vi "Intake Controller.vi"(8 "error in":errorcluster) -> ()   [LabVIEW 2020]
doc: "This VI executes continuously carrying out the current operation and responding to updates or new operations. It will often contain the timing or control code that is difficult to place directly in TeleOp. This VI generally opens all sensors and motors and isolates the rest of the robot code from knowing how the operations are carried out."
uses:
  <vilib>/Rock Robotics/WPI/Framework/Completion Status.ctl
  Intake Setpoints.ctl
  Intake Operations.ctl
  <vilib>/Rock Robotics/WPI/Solenoid/WPI_SolenoidValue.ctl
  <vilib>/Rock Robotics/WPI/Solenoid/WPI_SolenoidSetEnum.vi
  <vilib>/Rock Robotics/WPI/Solenoid/WPI_SolenoidGetEnum.vi
  <vilib>/Rock Robotics/Network Tables/NT Write Boolean.vi
panel:
  in  "Interactive Values":T1
  out "Current\nCmd":string
  in  "Buttons":cluster{"Execute Cmd":bool, "Abort Cmd":bool}
  out "Command Timing":cluster{"Start Time (ms)":u32, "Iterations":i32}
  out "Status":T3
  # "Tip: It may be helpful to observe inputs and sensor values.\nYou may also want to display tuning or debugging controls."
  # "Interactive Command: You may fill in the settings for a command\nand schedule it with the Execute button. You can observe and abort\nany command while fine tuning the code for the controller."
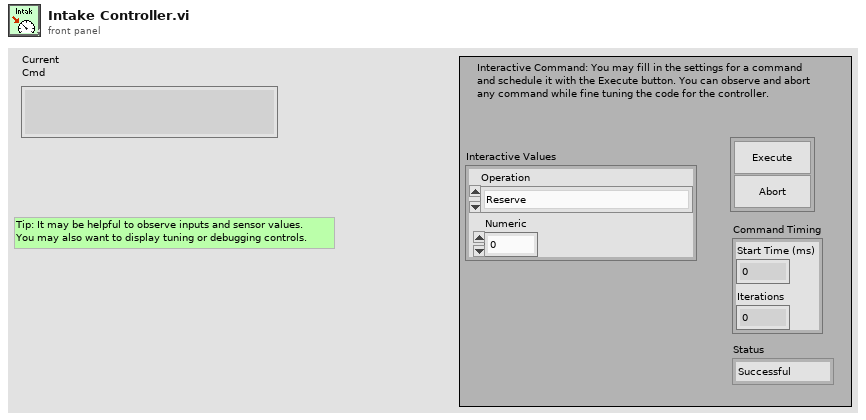
[diagram p1: front panel]
types:
  T1 = typedef "Intake Setpoints.ctl" = cluster{"Operation":T2, "Numeric":dbl}
  T2 = typedef "Intake Operations.ctl" = enum16{"Reserve", "Read Current", "Immediate", "Retract", "Extend", "Feed"}
  T3 = typedef "Completion Status.ctl" = enum16{"Successful", "Aborted", "Incomplete"}
  T4 = typedef "Command Status Info.ctl" = cluster{"Name":string, "Status":T3, "notifier out":T5}
  T5 = typedef "Completion Notifier.ctl" = refnum<notifier>
  T6 = cluster{"Current Command":T1, "Command Timing":cluster{"Start Time (ms)":u32, "Iterations":i32}, "Command Arguments":cluster{"Command Info":T4, "Description":string, "Default Command":T1, "queue out":refnum<queue>, "Subsystem Name":string}}
  T7 = typedef "WPI_SolenoidValue.ctl" = enum16{"Off", "On", "Forward", "Reverse"}
  T8 = typedef "WPI_SolenoidDevRef.ctl" = cluster{"DevStatus":errorcluster, "Pneumatics Control Module":u8, "Forward Solenoid Channel":T9, "Reverse Solenoid Channel":T9}
  T9 = typedef "WPI_SolenoidChannel.ctl" = enum8{"Solenoid 0", "Solenoid 1", "Solenoid 2", "Solenoid 3", "Solenoid 4", "Solenoid 5", "Solenoid 6", "Solenoid 7", "Solenoid 8", "Solenoid 9", "Solenoid 10", "Solenoid 11", "Solenoid 12", "Solenoid 13", "Solenoid 14", "Solenoid 15", "Invalid"}
  T10 = typedef "WPI_MotorControlDeviceRef.ctl" = cluster{"DeviceStatus":errorcluster, "Type":T11, "PWM":cluster{"PWM Channel":T12, "DeadBand":T13}, "CAN":cluster{"Device Number":u8, "SetOutput VI Ref":variant, "GetOutput VI Ref":variant, "Enable VI Ref":variant, "Disable VI Ref":variant, "Data":variant}, "Invert":bool, "DIO PWM":cluster{"PWM \"Enable\" Channel":T12, "DIOChannel":T14, "PWM Rate":dbl}}
  T11 = typedef "WPI_MotorControlType.ctl" = enum16{"PWM", "CAN", "DIO PWM"}
  T12 = typedef "FPGA_DIOPWMChannel.ctl" = enum8{"PWM 0", "PWM 1", "PWM 2", "PWM 3", "PWM 4", "PWM 5", "PWM 6", "PWM 7", "PWM 8", "PWM 9", "PWM MXP 0", "PWM MXP 1", "PWM MXP 2", "PWM MXP 3", "PWM MXP 4", "PWM MXP 5", "PWM MXP 6", "PWM MXP 7", "PWM MXP 8", "PWM MXP 9", "Invalid"}
  T13 = typedef "WPI_PWMDeadband.ctl" = cluster{"Name":string, "maxPositivePwm":i32, "minPositivePwm":i32, "centerPwm":i32, "maxNegativePwm":i32, "minNegativePwm":i32, "angularRange":u16}
  T14 = typedef "FPGA_DIOChannel.ctl" = enum8{"DIO 0", "DIO 1", "DIO 2", "DIO 3", "DIO 4", "DIO 5", "DIO 6", "DIO 7", "DIO 8", "DIO 9", "DIO MXP 0", "DIO MXP 1", "DIO MXP 2", "DIO MXP 3", "DIO MXP 4", "DIO MXP 5", "DIO MXP 6", "DIO MXP 7", "DIO MXP 8", "DIO MXP 9", "DIO MXP 10", "DIO MXP 11", "DIO MXP 12", "DIO MXP 13", "DIO MXP 14", "DIO MXP 15", "SPI Port CS1", "SPI Port CS2", "SPI Port CS3", "SPI Port MISO", "SPI Port MOSI", "Invalid"}
  T15 = typedef "WPI_DigitalInputDevRef.ctl" = cluster{"DevStatus":errorcluster, "DIO Channel":T14}
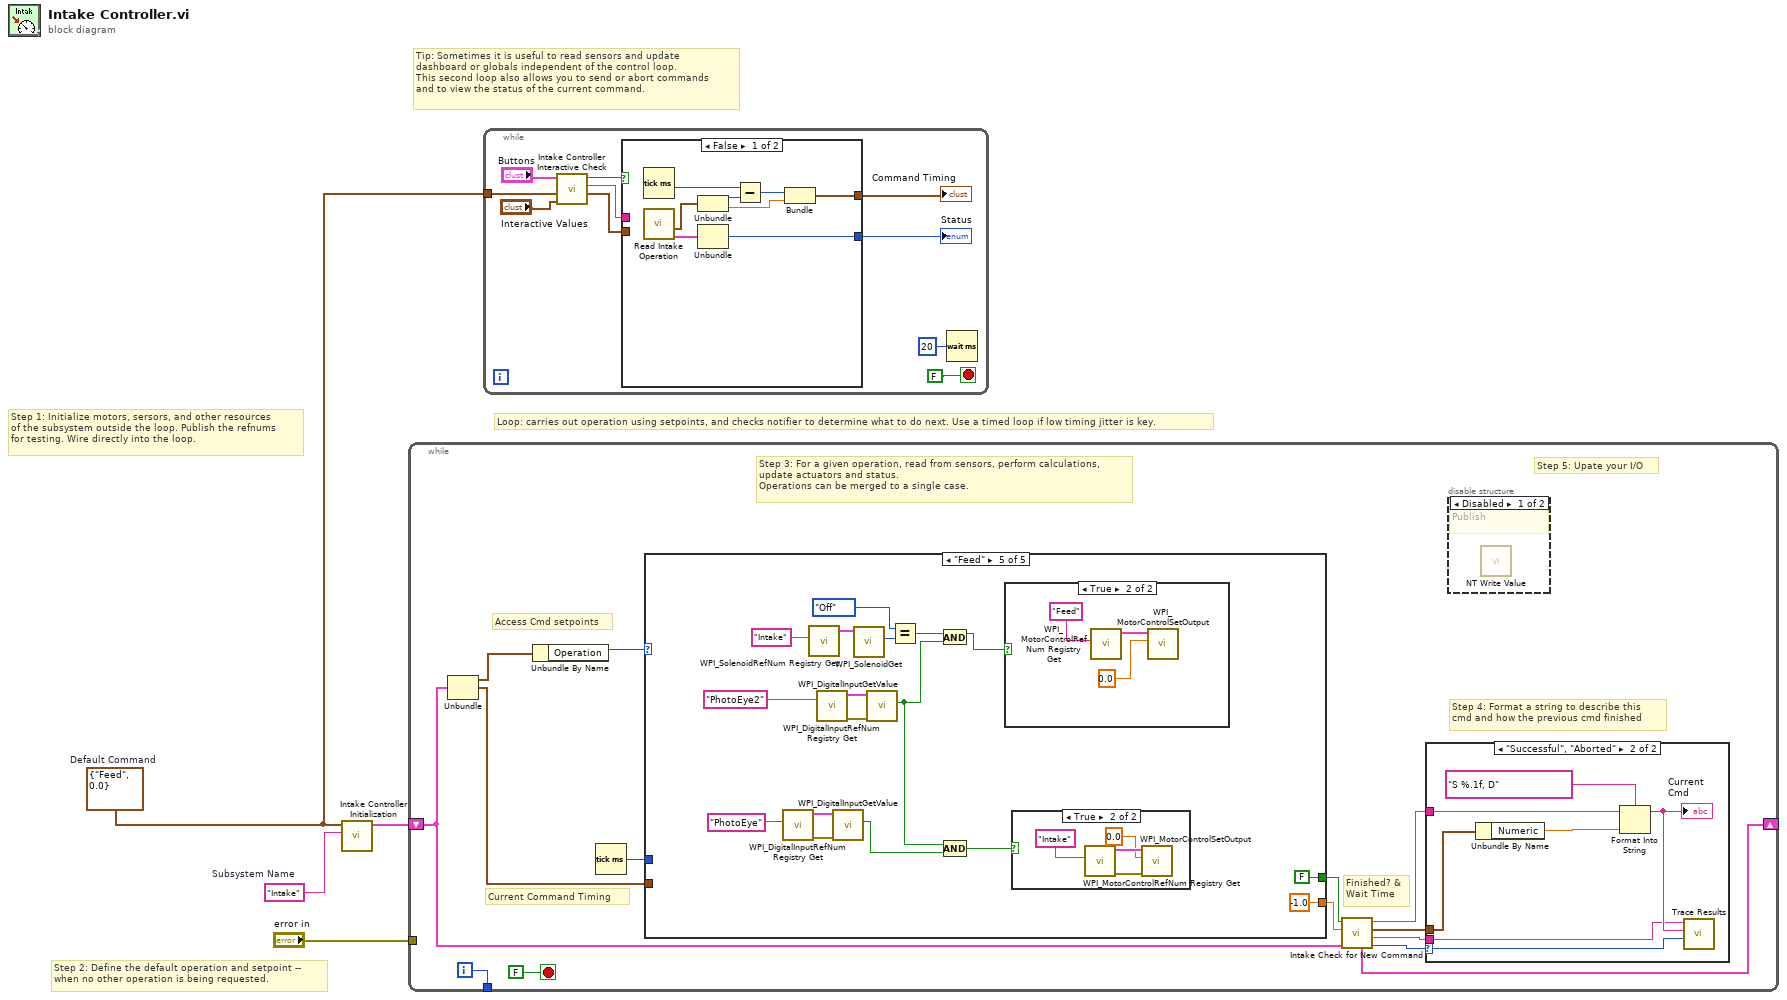
[diagram p0: block diagram]
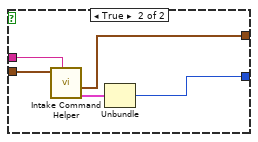
[diagram p2: hidden frame]
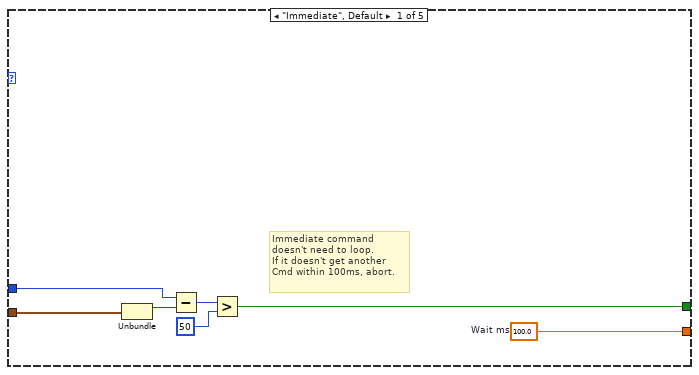
[diagram p5: hidden frame]
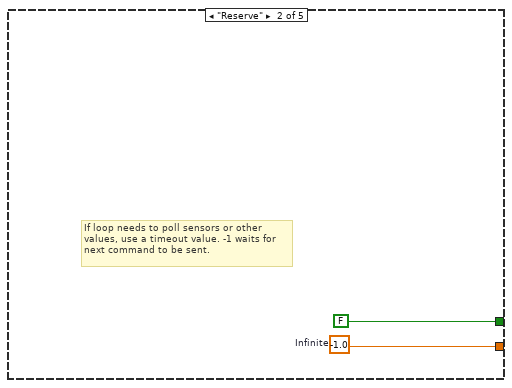
[diagram p6: hidden frame]
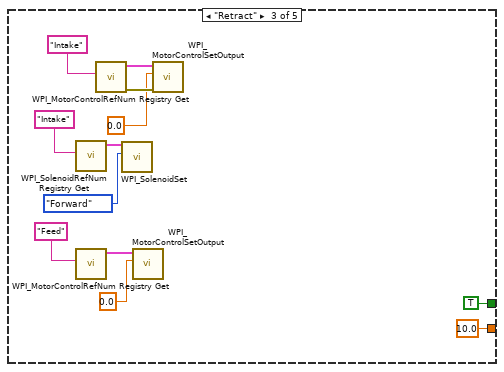
[diagram p7: hidden frame]
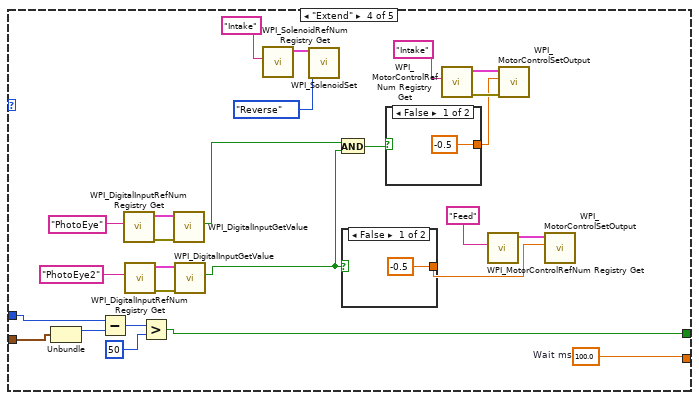
[diagram p8: hidden frame]
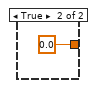
[diagram p9: hidden frame]
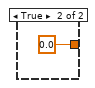
[diagram p10: hidden frame]
diagram:
  w1 = T1 {"Operation"=enum."Feed", "Numeric"=0.0}  # Default Command
  w2 = "Intake"  # Subsystem Name
  # "Tip: Sometimes it is useful to read sensors and update\ndashboard or globals independent of the control loop.\nThis second loop also allows you to send or abort commands\nand to view the status of the current command."
  # "Step 2: Define the default operation and setpoint --\nwhen no other operation is being requested."
  # "Step 1: Initialize motors, sersors, and other resources\nof the subsystem outside the loop. Publish the refnums\nfor testing. Wire directly into the loop."
  # "Loop: carries out operation using setpoints, and checks notifier to determine what to do next. Use a timed loop if low timing jitter is key."
  n1 = call "Intake Controller Initialization.vi"("Subsystem Name"=w2, "Default Command"=w1) -> ("Current Command"=w3:T6)  [unwired: 9 in]
  n2 = while {
    shift-right: [w12] -> _
    shift-left: w3 -> [w5]
    tunnel: [w17] -> _
    tunnel: "error in" -> [_]
    i -> [w17]
    stop <- FALSE stop-if-true
    # "Step 5: Upate your I/O"
    # "Step 4: Format a string to describe this\ncmd and how the previous cmd finished"
    # "Current Command Timing"
    # "Access Cmd setpoints"
    # "Finished? &\nWait Time"
    # "Step 3: For a given operation, read from sensors, perform calculations,\nupdate actuators and status.\nOperations can be merged to a single case."
    n3 = Unbundle(w5) -> ("Current Command"=w16:T1, "Command Timing"=w13:cluster{"Start Time (ms)":u32, "Iterations":i32})  [unwired: 1 out]
    n4 = Unbundle By Name(w16) -> ("Operation"=w15:T2)
    n5 = Tick Count (ms)() -> (millisecond timer value=w14:u32)
    n6 = case shown="\"Feed\"" w15 {
      tunnel: [w32 w34 10.0 ("Wait ms") w47 -1.0 ("Wait ms")] -> w10
      tunnel: [w26 FALSE ("ignore previous (F)") TRUE ("ignore previous (F)") w48 FALSE ("ignore previous (F)")] -> w11
      tunnel: w13 -> [w28 _ _ w49 _]
      tunnel: w14 -> [w27 _ _ w50 _]
      frame "Immediate", Default {
        w32 = 100.0  # Wait ms
        # "Immediate command\ndoesn't need to loop.\nIf it doesn't get another\nCmd within 100ms, abort."
        n7 = Unbundle(w28) -> ("Start Time (ms)"=w31:u32)  [unwired: 1 out]
        n8 = Subtract(x=w27, y=w31) -> (x-y=w30:u32)
        n9 = Greater?(x=w30, y=u8 50 ("Left Motor")) -> (0:w26:bool)
      }
      frame "Reserve" {
        w34 = -1.0  # Infinite
        # "If loop needs to poll sensors or other\nvalues, use a timeout value. -1 waits for\nnext command to be sent."
      }
      frame "Retract" {
        n10 = call <vilib>:"WPI_SolenoidRefNum Registry Get.vi"("refnum name"="Intake") -> ("SolenoidDevRef"=w45:T8)  [unwired: 9 in, 1 out]
        n11 = call <vilib>:"WPI_MotorControlRefNum Registry Get.vi"("refnum name"="Feed") -> ("MotorControlDevRef"=w46:T10)  [unwired: 9 in, 1 out]
        n12 = call <vilib>:"WPI_MotorControlRefNum Registry Get.vi"("refnum name"="Intake") -> ("error out"=w44:errorcluster, "MotorControlDevRef"=w43:T10)  [unwired: 9 in]
        n13 = call-poly <vilib>:"WPI_SolenoidSet.vi"("Value"=WPI_SolenoidValue."Forward", "SolenoidDevRef"=w45) -> ()  [unwired: 8 in, 2 out]
        n14 = call <vilib>:"WPI_MotorControlSetOutput.vi"("Output"=0.0, "MotorControlDevRef"=w46) -> ()  [unwired: 7 in, 3 out]
        n15 = call <vilib>:"WPI_MotorControlSetOutput.vi"("error in (no error)"=w44, "Output"=0.0, "MotorControlDevRef"=w43) -> ()  [unwired: 6 in, 3 out]
      }
      frame "Extend" {
        w47 = 100.0  # Wait ms
        n16 = Unbundle(w49) -> ("Start Time (ms)"=w53:u32)  [unwired: 1 out]
        n17 = Subtract(x=w50, y=w53) -> (x-y=w52:u32)
        n18 = call <vilib>:"WPI_DigitalInputRefNum Registry Get.vi"("refnum name"="PhotoEye") -> ("error out"=w63:errorcluster, "DigitalInputDevRef"=w62:T15)  [unwired: 9 in]
        n19 = call <vilib>:"WPI_DigitalInputRefNum Registry Get.vi"("refnum name"="PhotoEye2") -> ("error out"=w61:errorcluster, "DigitalInputDevRef"=w60:T15)  [unwired: 9 in]
        n20 = Greater?(x=w52, y=u8 50 ("Left Motor")) -> (0:w48:bool)
        n21 = call <vilib>:"WPI_DigitalInputGetValue.vi"("error in (no error)"=w63, "DigitalInputDevRef"=w62) -> ("Value"=w57:bool)  [unwired: 7 in, 2 out]
        n22 = call <vilib>:"WPI_DigitalInputGetValue.vi"("error in (no error)"=w61, "DigitalInputDevRef"=w60) -> ("Value"=w56:bool)  [unwired: 7 in, 2 out]
        n23 = call <vilib>:"WPI_SolenoidRefNum Registry Get.vi"("refnum name"="Intake") -> ("SolenoidDevRef"=w72:T8)  [unwired: 9 in, 1 out]
        n24 = call-poly <vilib>:"WPI_SolenoidSet.vi"("Value"=WPI_SolenoidValue."Reverse", "SolenoidDevRef"=w72) -> ()  [unwired: 8 in, 2 out]
        n25 = And(x=w57, y=w56) -> (x .and. y?=w66:bool)
        n26 = case shown="False" w56 {
          tunnel: [-0.5 ("Output") 0.0 ("Output")] -> w55
          frame False {
          }
          frame True {
          }
        }
        n27 = case shown="False" w66 {
          tunnel: [-0.5 ("Output") 0.0 ("Output")] -> w54
          frame False {
          }
          frame True {
          }
        }
        n28 = call <vilib>:"WPI_MotorControlRefNum Registry Get.vi"("refnum name"="Intake") -> ("error out"=w68:errorcluster, "MotorControlDevRef"=w67:T10)  [unwired: 9 in]
        n29 = call <vilib>:"WPI_MotorControlRefNum Registry Get.vi"("refnum name"="Feed") -> ("MotorControlDevRef"=w65:T10)  [unwired: 9 in, 1 out]
        n30 = call <vilib>:"WPI_MotorControlSetOutput.vi"("error in (no error)"=w68, "Output"=w54, "MotorControlDevRef"=w67) -> ()  [unwired: 6 in, 3 out]
        n31 = call <vilib>:"WPI_MotorControlSetOutput.vi"("Output"=w55, "MotorControlDevRef"=w65) -> ()  [unwired: 7 in, 3 out]
      }
      frame "Feed" {
        n32 = call <vilib>:"WPI_DigitalInputRefNum Registry Get.vi"("refnum name"="PhotoEye") -> ("error out"=w83:errorcluster, "DigitalInputDevRef"=w82:T15)  [unwired: 9 in]
        n33 = call <vilib>:"WPI_SolenoidRefNum Registry Get.vi"("refnum name"="Intake") -> ("SolenoidDevRef"=w92:T8)  [unwired: 9 in, 1 out]
        n34 = call <vilib>:"WPI_DigitalInputRefNum Registry Get.vi"("refnum name"="PhotoEye2") -> ("error out"=w88:errorcluster, "DigitalInputDevRef"=w87:T15)  [unwired: 9 in]
        n35 = call <vilib>:"WPI_DigitalInputGetValue.vi"("error in (no error)"=w83, "DigitalInputDevRef"=w82) -> ("Value"=w80:bool)  [unwired: 7 in, 2 out]
        n36 = call-poly <vilib>:"WPI_SolenoidGet.vi"("SolenoidDevRef"=w92) -> ("Value"=w93:T7)  [unwired: 8 in, 2 out]
        n37 = call <vilib>:"WPI_DigitalInputGetValue.vi"("error in (no error)"=w88, "DigitalInputDevRef"=w87) -> ("Value"=w79:bool)  [unwired: 7 in, 2 out]
        n38 = Equal?(x=WPI_SolenoidValue."Off", y=w93) -> (x = y?=w78:bool)
        n39 = And(x=w78, y=w79) -> (x .and. y?=w89:bool)
        n40 = Compound Arithmetic op=AND(w79, w80) -> (w77:bool)
        n41 = case shown="True" w89 {
          frame False {
          }
          frame True {
            n42 = call <vilib>:"WPI_MotorControlRefNum Registry Get.vi"("refnum name"="Feed") -> ("MotorControlDevRef"=w100:T10)  [unwired: 9 in, 1 out]
            n43 = call <vilib>:"WPI_MotorControlSetOutput.vi"("Output"=0.0, "MotorControlDevRef"=w100) -> ()  [unwired: 7 in, 3 out]
          }
        }
        n44 = case shown="True" w77 {
          frame False {
          }
          frame True {
            n45 = call <vilib>:"WPI_MotorControlRefNum Registry Get.vi"("refnum name"="Intake") -> ("error out"=w96:errorcluster, "MotorControlDevRef"=w97:T10)  [unwired: 9 in]
            n46 = call <vilib>:"WPI_MotorControlSetOutput.vi"("error in (no error)"=w96, "Output"=0.0, "MotorControlDevRef"=w97) -> ()  [unwired: 6 in, 3 out]
          }
        }
      }
    }
    n47 = call "Intake Check for New Command.vi"("Current Command"=w5, "Wait time (ms)"=w10, "Finished?"=w11) -> ("Completion"=w6:T3, "Subsystem Name"=w7:string, "Current Command"=w8:T1, "Initial Trace String"=w9:string, "NextCommand"=w12:T6)  [unwired: 4 in]
    n48 = case shown="\"Successful\", \"Aborted\"" w6 {
      selector: w6 -> [_ w25]
      tunnel: w9 -> [_ w21]
      tunnel: w8 -> [_ w22]
      tunnel: w7 -> [_ w19]
      frame "Incomplete", Default {
        # "Continuing current command"
      }
      frame "Successful", "Aborted" {
        # "Report and setup for next command"
        n49 = Unbundle By Name(w22) -> ("Numeric"=w24:dbl)
        n50 = Format Into String(format string="S %.1f, D", initial string=w21, w24) -> (resulting string=w20:string)  [unwired: 1 in, 1 out]
        "Current\nCmd" <- w20
        n51 = call <vilib>:"Trace Results.vi"("Status of previous command"=w25, "Description"=w20, "Subsystem"=w19) -> ()  [unwired: 9 in]
      }
    }
    n52 = disable-structure shown="Disabled" {
      frame Disabled {
        # "Publish"
        n53 = call-poly <vilib>:"NT Write Value.vi"() -> ()  [unwired: 11 in, 1 out]
      }
      frame Enabled {
      }
    }
  }
  n54 = while {
    tunnel: w1 -> [w107]
    stop <- FALSE stop-if-true
    n55 = call "Intake Controller Interactive Check.vi"("Interactive Command in"="Interactive Values", "Default Command"=w107, "Buttons"="Buttons") -> ("Interactive Command out"=w104:T1, "Trace String"=w105:string, "Schedule"=w106:bool)  [unwired: 6 in]
    n56 = case shown="False" w106 {
      tunnel: [w118 w123] -> w103
      tunnel: w104 -> [_ w121]
      tunnel: [w111 w119] -> w102
      tunnel: w105 -> [_ w122]
      frame False {
        n57 = Tick Count (ms)() -> (millisecond timer value=w114:u32)
        n58 = call "Read Intake Operation.vi"() -> ("Command Info"=w112:T4, "SubSystem Data"=w113:T1)  [unwired: 9 in, 1 out]
        n59 = Unbundle(w113) -> ("Operation"=w117:T2, "Numeric"=w115:dbl)
        n60 = Unbundle(w112) -> ("Status"=w118:T3)  [unwired: 2 out]
        n61 = Subtract(x=w114, y=w117) -> (x-y=w116:u32)
        n62 = Bundle(w116, "Numeric"=w115) -> (w111:cluster{u32, "Numeric":dbl})  [unwired: 1 in]
      }
      frame True {
        n63 = call "Intake Command Helper.vi"("Description"=w122, "SubSystem Data"=w121) -> ("Command Info Out"=w120:T4, "Command Timing"=w119:cluster{"Start Time (ms)":u32, "Iterations":i32})  [unwired: 7 in, 1 out]
        n64 = Unbundle(w120) -> ("Status"=w123:T3)  [unwired: 2 out]
      }
    }
    "Status" <- w103
    "Command Timing" <- w102
    n65 = Wait (ms)(milliseconds to wait=u32 20) -> ()  [unwired: 1 out]
  }
